vi "ReportHead.vi"(8 "error in (no error)":errorcluster caption="错误输入（无错误）", 11 "产品状态":string) -> (0 "error out":errorcluster caption="错误输出", 3 "report out":refnum<class "NI_report.lvclass"> caption="报表输出")   [LabVIEW 2020]
uses:
  <vilib>/Utility/NIReport.llb/NI_report.lvclass
  <vilib>/addons/_office/_exclsub.llb/font.ctl
  <vilib>/Utility/NIReport.llb/Report Type.ctl
  Global_Variable/Global.vi
  <vilib>/Utility/NIReport.llb/Append Report Text (str wrap).vi
  <vilib>/addons/_office/NI_ReportGenerationToolkit.lvlib
  <vilib>/Utility/NIReport.llb/NI_ReportGenerationCore.lvlib
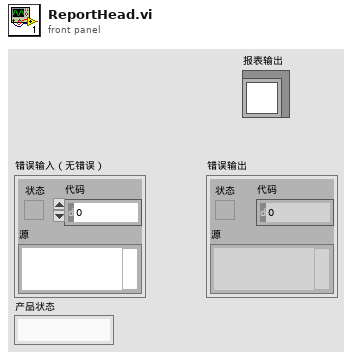
[diagram p1: front panel]
types:
  T1 = typedef "NI_ReportGenerationCore.lvlib/Report Type.ctl" = enum16{"HTML", "Word", "Excel"}
  T2 = enum16{"maximized", "minimized", "normal", "no change"}
  T3 = cluster{"操作者编号":string, "操作者姓名":string, "操作者权限":string, "联机状态":string, "产品型号":string, "产品状态":string}
  T4 = cluster{"top":dbl, "left":dbl, "right":dbl, "bottom":dbl}
  T5 = cluster{"Charset (-1)":i16, "Weight (-1)":i16, "Name":string, "Size":string}
  T6 = cluster{"Italic":enum16{"Italic Unchanged", "Italic On", "Italic Off"}, "Strike Through":enum16{"Strike Through Unchanged", "Strike Through On", "Strike Through Off"}, "Underline":enum16{"Underline Unchanged", "Underline On", "Underline Off"}, "Bold":enum16{"Bold Unchanged", "Bold On", "Bold Off"}}
  T7 = typedef "NI_ReportGenerationToolkit.lvlib/font.ctl" = cluster{"font name":string, "font size":dbl, "bold":u16, "italic":u16, "underline":u16, "strike through":u16, "font color":u32}
  T8 = cluster{"用户编号":string, "用户名":string, "用户密码(密文)":string, "用户权限":string}
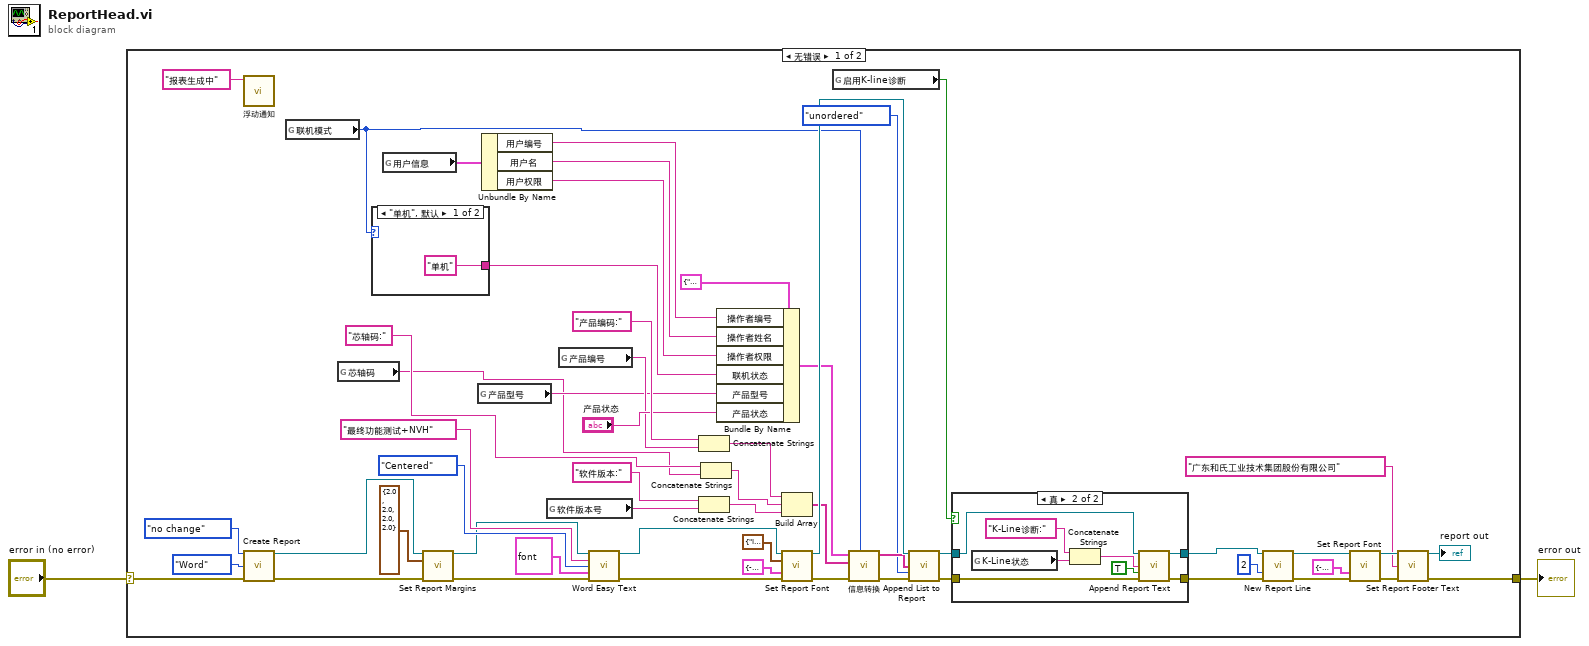
[diagram p0: block diagram]
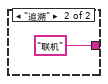
[diagram p3: hidden frame]
diagram:
  n1 = case shown="无错误" "error in (no error)" {
    selector: "error in (no error)" -> [w36 w70]
    tunnel: [w32 w70] -> w1
    frame No Error {
      n2 = call "浮动通知.vi"("通知内容"="报表生成中" ("Status")) -> ()  [unwired: 11 in]
      n3 = call <vilib>:"Create Report.vi"("window state (normal)"=T2."no change", "report type"=Report_Type."Word", "error in (no error)"=w36) -> ("report out"=w47:refnum<class "NI_report.lvclass">, "error out"=w44:errorcluster)  [unwired: 11 in]
      n4 = global read "Global.vi" "联机模式"() -> (w14:enum16{"单机", "追溯"})
      n5 = global read "Global.vi" "芯轴码"() -> (w3:string)
      n6 = case shown="\"单机\", 默认" w14 {
        tunnel: ["单机" "联机"] -> w30
        frame "单机", Default {
        }
        frame "追溯" {
        }
      }
      n7 = global read "Global.vi" "用户信息"() -> (w18:T8)
      n8 = call-dynamic "Set Report Margins.vi"("report in"=w47, "margins (1.00)"=T4 {"top"=2.0, "left"=2.0, "right"=2.0, "bottom"=2.0}, "error in (no error)"=w44) -> ("report out"=w46:refnum<class "NI_report.lvclass">, "error out"=w45:errorcluster)  [unwired: 10 in, 1 out]
      n9 = global read "Global.vi" "产品型号"() -> (w21:string)
      n10 = Unbundle By Name(w18) -> ("用户编号"=w17:string, "用户名"=w16:string, "用户权限"=w15:string)
      n11 = global read "Global.vi" "软件版本号"() -> (w7:string)
      n12 = global read "Global.vi" "产品编号"() -> (w22:string)
      n13 = call <vilib>:"Word Easy Text.vi"("report in"=w46, "text"="最终功能测试+NVH", "alignment (left)"=enum16{"Left", "Centered", "Right", "Justify"}."Centered", "font"=T7 {"font name"="楷体", "font size"=26.0, "bold"=1, "italic"=2, "underline"=2, "strike through"=2, "font color"=16777228}, "error in (no error)"=w45) -> ("report out"=w55:refnum<class "NI_report.lvclass">, "error out"=w54:errorcluster)  [unwired: 8 in, 1 out]
      n14 = Concatenate Strings("产品编码:", w22) -> (w26:string)
      n15 = Concatenate Strings("软件版本:", w7) -> (w6:string)
      n16 = Concatenate Strings("芯轴码:", w3) -> (w5:string)
      n17 = Bundle By Name(cluster=T3 {"操作者编号"="001", "操作者姓名"="Administrator", "操作者权限"="系统管理员", "联机状态"="单机", "产品型号"="SL7202", "产品状态"=""} ("测试信息"), "操作者编号"=w17, "操作者姓名"=w16, "操作者权限"=w15, "联机状态"=w30, "产品型号"=w21, "产品状态"="产品状态") -> (w28:T3)
      n18 = Build Array(w26, w5, w6) -> (w25:string[])
      n19 = call-dynamic "Set Report Font.vi"("report in"=w55, "text options"=T6 {"Italic"=enum."Italic Off", "Strike Through"=enum."Strike Through Unchanged", "Underline"=enum."Underline Off", "Bold"=enum."Bold Off"}, "font settings"=T5 {"Charset (-1)"=-1, "Weight (-1)"=-1, "Name"="微软雅黑 Light", "Size"="12 "}, "error in (no error)"=w54) -> ("report out"=w42:refnum<class "NI_report.lvclass">, "error out"=w35:errorcluster)  [unwired: 9 in, 1 out]
      n20 = global read "Global.vi" "启用K-line诊断"() -> (w13:bool)
      n21 = call "信息转换.vi"("联机模式"=w14, "错误输入（无错误）"=w35, "追溯码"=w25, "测试信息"=w28) -> ("错误输出"=w34:errorcluster, "信息输出"=w37:string[])  [unwired: 6 in]
      n22 = call-dynamic "Append List to Report.vi"("report in"=w42, "list elements"=w37, "list type (ordered)"=enum16{"unordered", "ordered"}."unordered", "error in (no error)"=w34) -> ("report out"=w12:refnum<class "NI_report.lvclass">, "error out"=w11:errorcluster)  [unwired: 8 in, 2 out]
      n23 = case shown="真" w13 {
        tunnel: w12 -> [w59 w64]
        tunnel: w11 -> [w58 w62]
        tunnel: [w59 w61] -> w10
        tunnel: [w58 w60] -> w9
        frame False {
        }
        frame True {
          n24 = global read "Global.vi" "K-Line状态"() -> (w66:string)
          n25 = Concatenate Strings("K-Line诊断:" ("text"), w66) -> (w65:string)
          n26 = call-poly <vilib>:"Append Report Text.vi"("report in"=w64, "text"=w65, "append on new line? (F)"=TRUE, "error in (no error)"=w62) -> ("report out"=w61:refnum<class "NI_report.lvclass">, "error out"=w60:errorcluster)  [unwired: 8 in, 2 out]
        }
      }
      n27 = call-dynamic "New Report Line.vi"("report in"=w10, "number of lines (1)"=2, "error in (no error)"=w9) -> ("report out"=w40:refnum<class "NI_report.lvclass">, "error out"=w41:errorcluster)  [unwired: 11 in]
      n28 = call-dynamic "Set Report Font.vi"("report in"=w40, "font settings"=T5 {"Charset (-1)"=-1, "Weight (-1)"=-1, "Name"="楷体", "Size"="9 "}, "error in (no error)"=w41) -> ("report out"=w51:refnum<class "NI_report.lvclass">, "error out"=w50:errorcluster)  [unwired: 10 in, 1 out]
      n29 = call-dynamic "Set Report Footer Text.vi"("report in"=w51, "center footer text"="广东和氏工业技术集团股份有限公司", "error in (no error)"=w50) -> ("report out"=→"report out":refnum<class "NI_report.lvclass">, "error out"=w32:errorcluster)  [unwired: 11 in]
    }
    frame Error {
    }
  }
  "error out" <- w1
